vi "Main_v4.vi"() -> ()   [LabVIEW 2020]
uses:
  <userlib>/LevyLab/Relay Box/Type_defs/Resistor--enum.ctl
  <vilib>/Analysis/Matrix/Datatypes/RealMatrix.ctl
  subVIs/Global Variables.vi
  <vilib>/picture/3D Picture Control/Helpers/Apply Texture (no reference).vi
  <vilib>/picture/3D Picture Control/NI_3D Picture Control.lvlib
  <vilib>/Analysis/Matrix/NI_Matrix.lvlib
panel:
  in  "Run 2":bool=TRUE
  in  "Refresh Button":bool
  out "Ready?":bool
  in  "Done":bool
  in  "Help":bool
  in  "Abort":bool
  in  "Run":bool
  out "Estimated Time\nfor Lithography":timestamp=timestamp(-68372.87678205769 s since 1904-01-01) format="%<%H:%M:%S>T"
  in  "Visualization":T1(tab)
  out "Render":T2(plugin-control)
  out "Voltage Mapping":dbl(ramp)
  out "2D":T2(plugin-control)
  out "3D Picture":refnum<vi>(3d-picture)
  in  "Settings":T3(tab)
  in  "interpolation distance":dbl=0.1
  in  "Lithography Config File (.lcf)":path=path "c:/"
  in  "Patterns (drag-and-drop reorder)":i32(listbox)
  in  "image data max":dbl(slide)=100.0 min=0.0 max=100.0 scale=0.0..100.0
  in  "image data min":dbl(slide)=17.365269461077844 min=0.0 max=100.0 scale=0.0..100.0
  in  "AFM Type":u16(ring)=1 items=["Cypher", "MFP3D", "MFP3D_Lucy", "Simulation"]
  in  "Page":i32=1 min=0
  in  "Inkscape File (.svg)":path=path "c:/"
  in  "Background Image":path=path "c:/"
  # "Before you start the program\nchange these paths to the\ncorresponding files"
  # "In simulation mode, to change the perspective, hold the left button of mouse and drag in the picture.\nTo zoom in and out, hold the shift button, hold the left button of the mouse and drag up and down in\nthe picture."
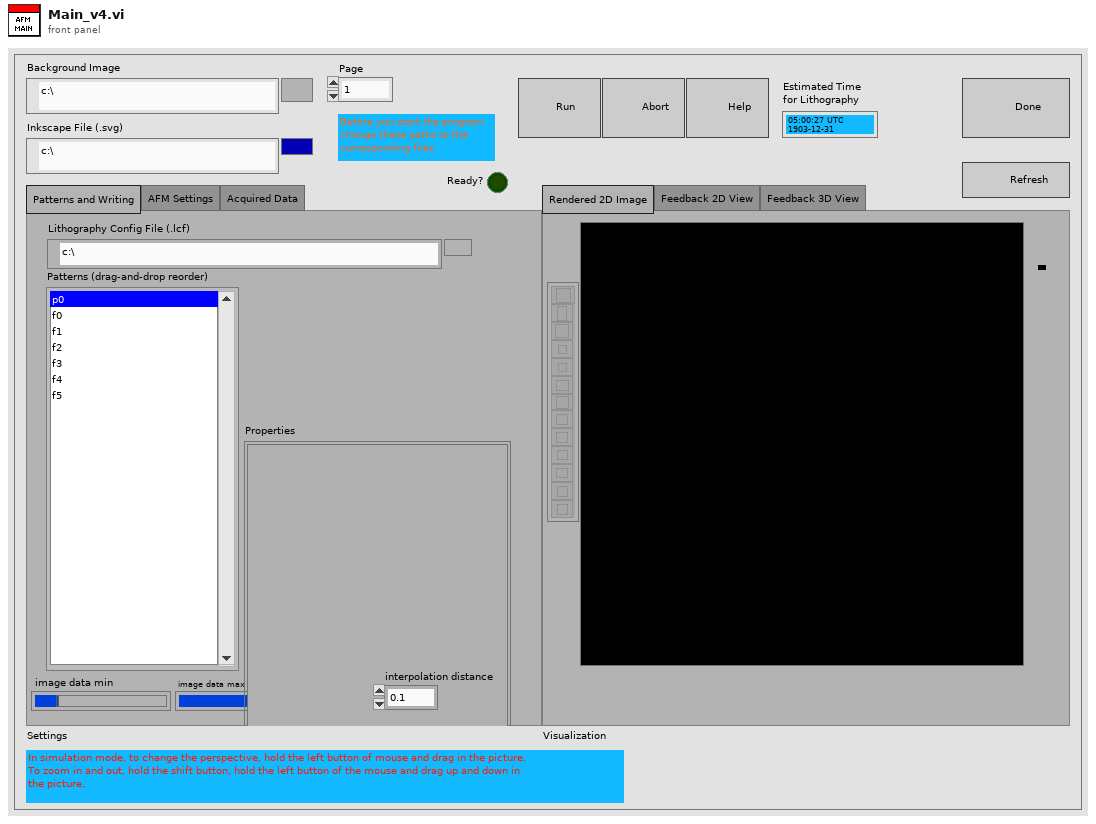
[diagram p1: front panel]
types:
  T1 = enum32{"Rendered 2D Image", "Feedback 2D View", "Feedback 3D View"}
  T2 = typedef "IMAQ Image.ctl" = refnum<image>
  T3 = enum32{"Patterns and Writing", "AFM Settings", "Acquired Data"}
  T4 = enum32{"invalid app kind", "Development System", "Run Time System", "Student Edition", "Embedded LabVIEW", "Evaluation", "Custom"}
  T5 = enum32{"Invalid", "Standard", "Closed", "Hidden", "Minimized", "Maximized"}
  T6 = typedef "Rectangle Properties - cluster.ctl" = cluster{"Enabled":bool, "Direction":u16, "Fill Orientation":u16, "Fill Spacing":dbl, "Speed (um/s)":T7, "Voltage (V)":T7, "Set Resistance":T10}
  T7 = typedef "Voltage - cluster.ctl" = cluster{"Schedule":T8, "Value":dbl, "Start Value":dbl, "End Value":dbl, "Min Value":dbl, "Max Value":dbl, "Duty Cycle (%)":dbl, "Signal Type":T9, "Cycle Number":dbl, "Phase (degrees)":dbl, "formula":string, "formula length (nm)":dbl, "formula resolution (nm)":dbl}
  T8 = typedef "Schedule - enum.ctl" = enum16{"Constant", "Ramp", "Fn. Generator", "Formula"}
  T9 = typedef "Signal Type - enum.ctl" = enum16{"Sine Wave", "Triangle Wave", "Square Wave", "Sawtooth Wave"}
  T10 = typedef "Resistor--enum.ctl" = enum16{"open", "discharge tip", "0 ohms", "100k ohm", "10M ohm", "1G ohm"}
  T11 = typedef "Funnel Properties - cluster.ctl" = cluster{"Enabled":bool, "Direction":u16, "Smooth Segments":dbl, "Bottom Segs.":dbl, "Speed (um/s)":T7, "Voltage (V)":T7, "Set Resistance":T10}
  T12 = typedef "Path Properties - cluster.ctl" = cluster{"Enabled":bool, "Direction":u16, "Fill Orientation":u16, "Smooth Segments":dbl, "Fill Spacing":dbl, "Speed (um/s)":T7, "Voltage (V)":T7, "Set Resistance":T10}
  T13 = cluster{"Path Properties":T12[], "Rectangle Properties":T6[], "Funnel Properties":T11[]}
  T14 = cluster{"SceneObject out":refnum<vi>, "Tip":refnum<vi>, "Canvas":refnum<vi>}
  T15 = typedef "imagedata.ctl" = cluster{"image type":i32, "image depth":i32, "image":u8[], "mask":u8[], "colors":u32[], "Rectangle":cluster{"left":i16, "top":i16, "right":i16, "bottom":i16}}
  T16 = typedef "NI_Matrix.lvlib/RealMatrix.ctl" = dbl[][]
  T17 = cluster{"Core":cluster{"Current VI Reference":refnum<vi>, "Close Panel on Exit?":bool}, "Parsing Data":cluster{"paths":cluster{"Fill Color":string, "Stroke Color":string, "Commands":cluster{"Command Type":string, "Coordinates":cluster{"X":dbl, "Y":dbl}[]}[], "Transformation Matrix 2":T16}[], "funnels":cluster{"Fill Color":string, "Stroke Color":string, "Commands":cluster{"Command Type":string, "Coordinates":cluster{"X":dbl, "Y":dbl}[]}[], "Transformation Matrix 2":T16}[], "rects":cluster{"Fill Color":string, "Stroke Color":string, "Width":dbl, "Height":dbl, "X":dbl, "Y":dbl, "Transformation Matrix":T16}[]}, "Lithography Data":cluster{"Name":string, "Litho":cluster{"X":dbl, "Y":dbl, "Speed":dbl, "Voltage":dbl}[], "Set Resistance":T10}[], "VI Refs":refnum<vi>[], "Data Queue":refnum<queue>, "3D":cluster{"SceneObject out":refnum<vi>, "Tip":refnum<vi>, "Canvas":refnum<vi>}}
  T18 = cluster{"paths":cluster{"Fill Color":string, "Stroke Color":string, "Commands":cluster{"Command Type":string, "Coordinates":cluster{"X":dbl, "Y":dbl}[]}[], "Transformation Matrix 2":T16}[], "funnels":cluster{"Fill Color":string, "Stroke Color":string, "Commands":cluster{"Command Type":string, "Coordinates":cluster{"X":dbl, "Y":dbl}[]}[], "Transformation Matrix 2":T16}[], "rects":cluster{"Fill Color":string, "Stroke Color":string, "Width":dbl, "Height":dbl, "X":dbl, "Y":dbl, "Transformation Matrix":T16}[]}
  T19 = cluster{"Name":string, "Litho":cluster{"X":dbl, "Y":dbl, "Speed":dbl, "Voltage":dbl}[], "Set Resistance":T10}[]
  T20 = cluster{"Current VI Reference":refnum<vi>, "Close Panel on Exit?":bool}
  T21 = cluster{"X":dbl, "Y":dbl, "Speed":dbl, "Voltage":dbl}
  T22 = cluster{" paths":cluster{"Fill Color":string, "Stroke Color":string, "Commands":cluster{"Command Type":string, "Coordinates":cluster{"X":dbl, "Y":dbl}[]}[], "Transformation Matrix 2":T16}[], " funnels":cluster{"Fill Color":string, "Stroke Color":string, "Commands":cluster{"Command Type":string, "Coordinates":cluster{"X":dbl, "Y":dbl}[]}[], "Transformation Matrix 2":T16}[], "rects":cluster{"Fill":string, "Stroke":string, "width":dbl, "height":dbl, "x":dbl, "y":dbl, "Transformation Matrix":T16}[]}
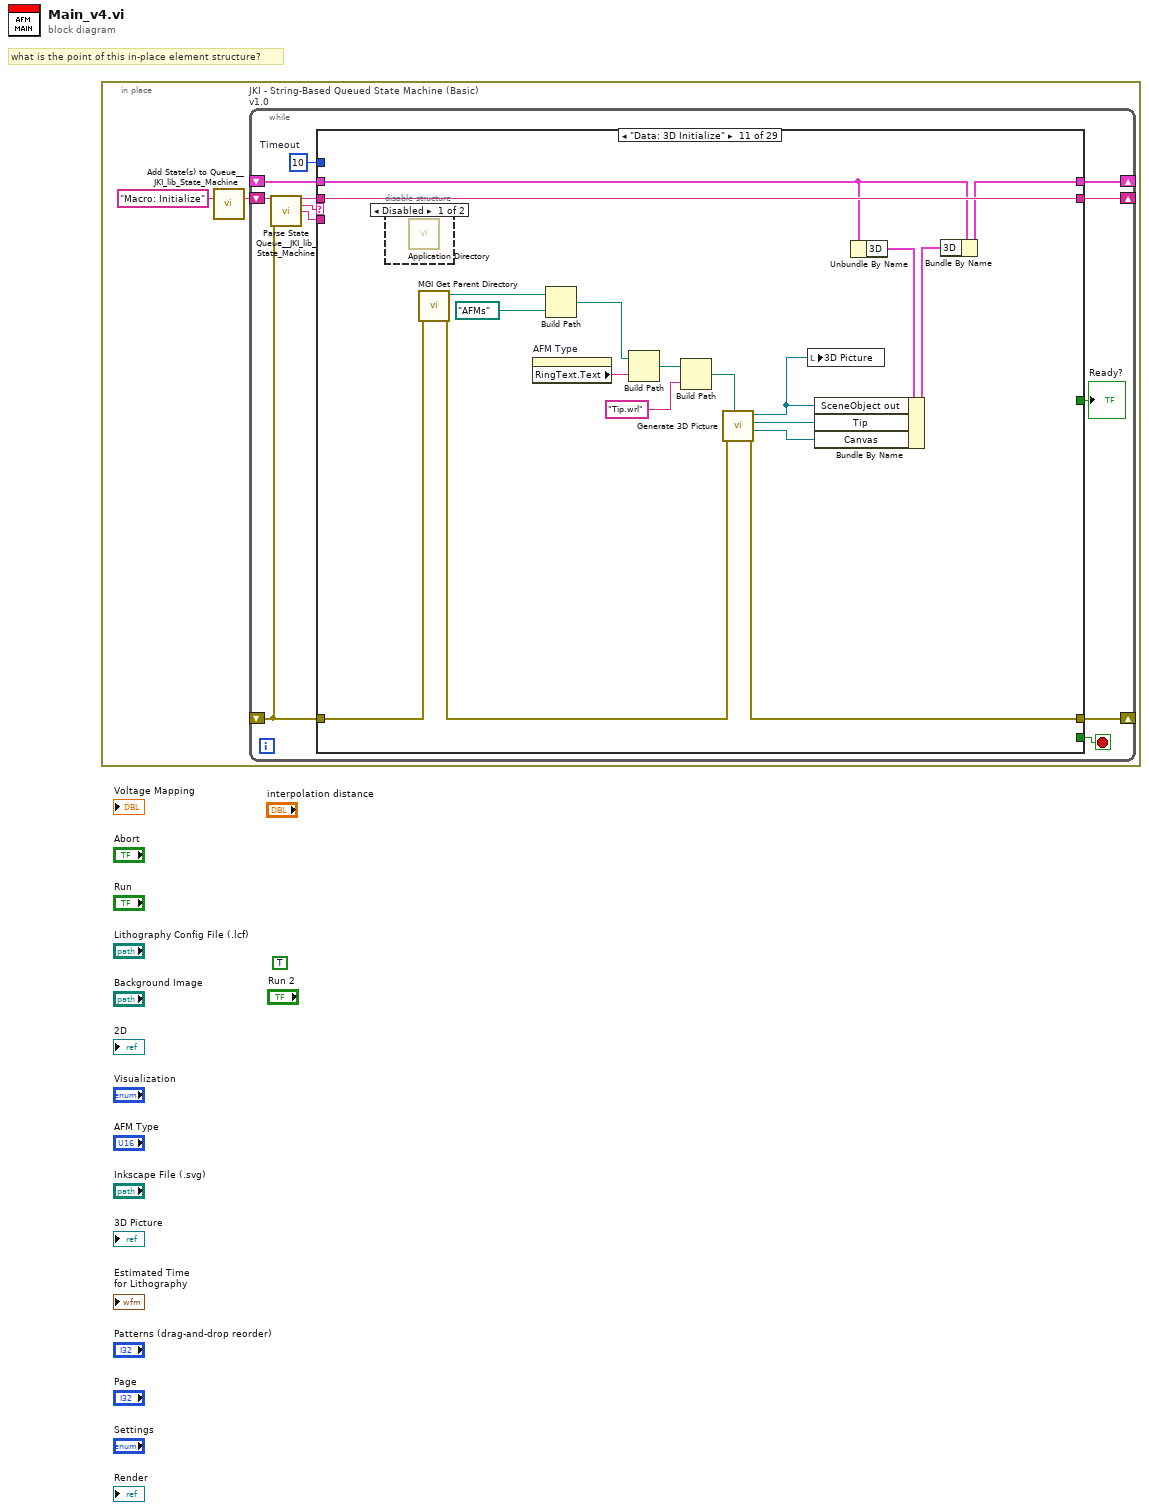
[diagram p0: block diagram]
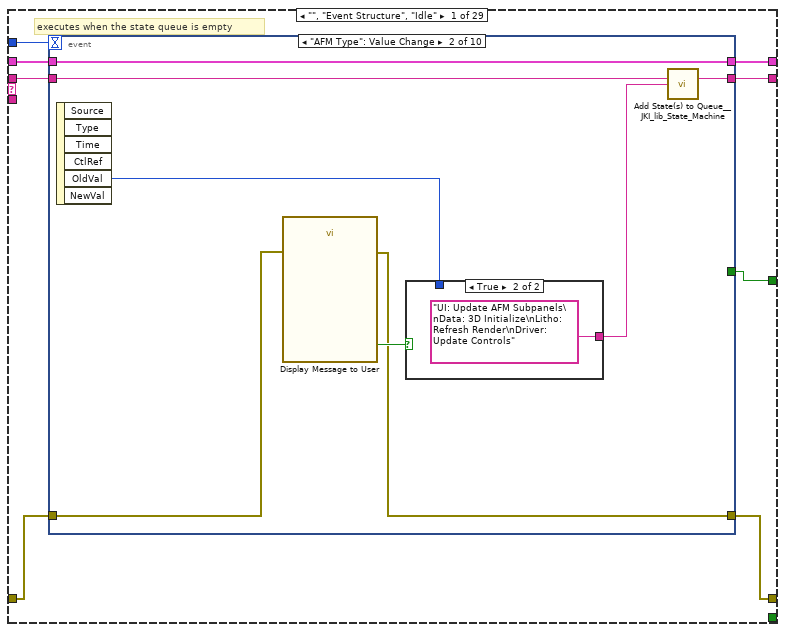
[diagram p2: hidden frame]
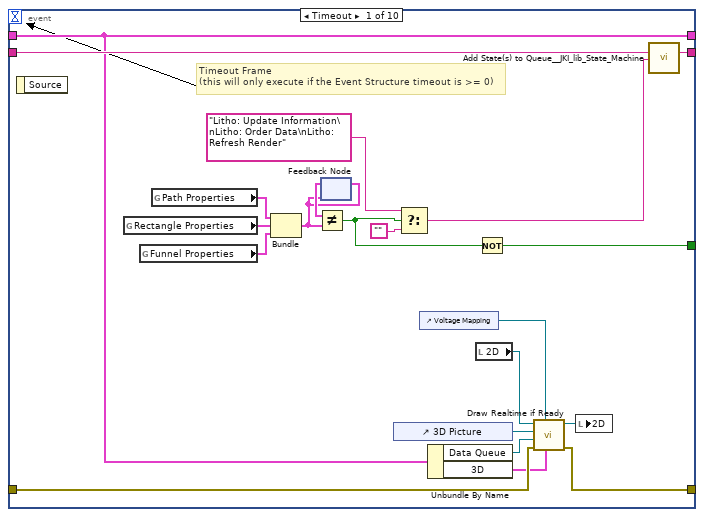
[diagram p3: hidden frame]
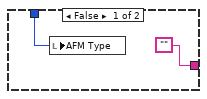
[diagram p4: hidden frame]
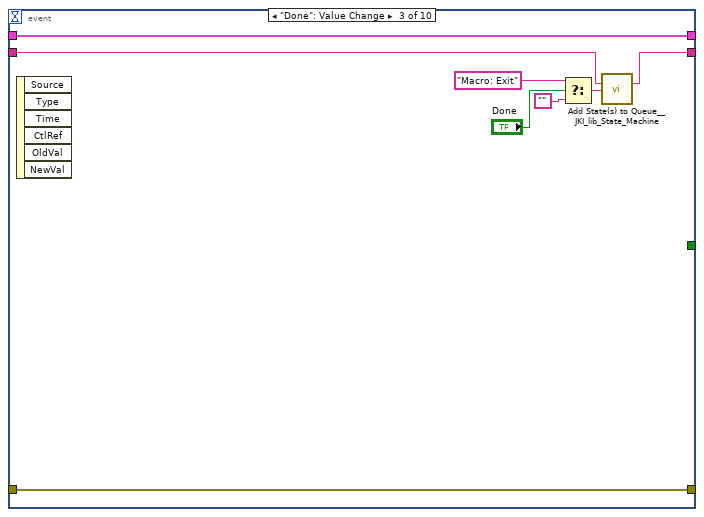
[diagram p5: hidden frame]
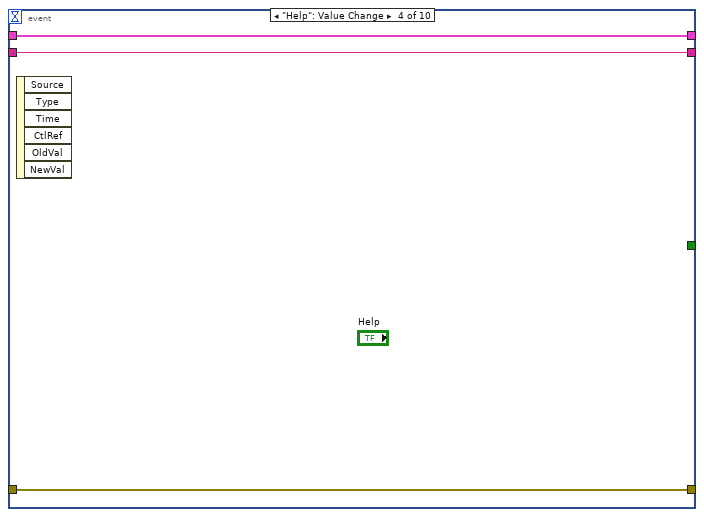
[diagram p6: hidden frame]
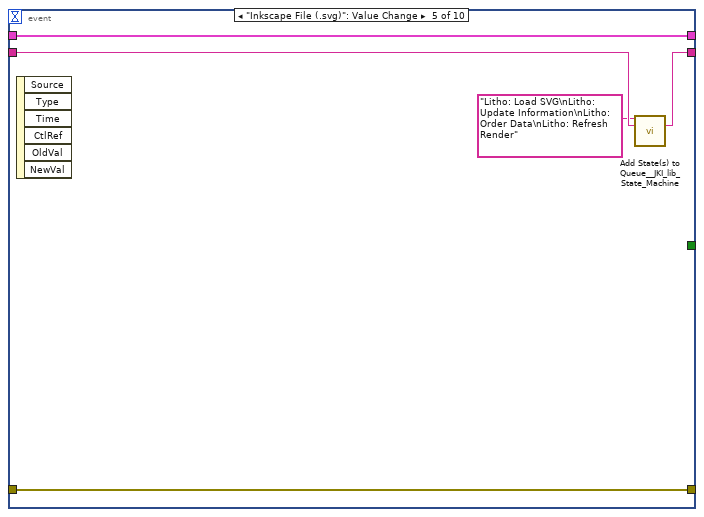
[diagram p7: hidden frame]
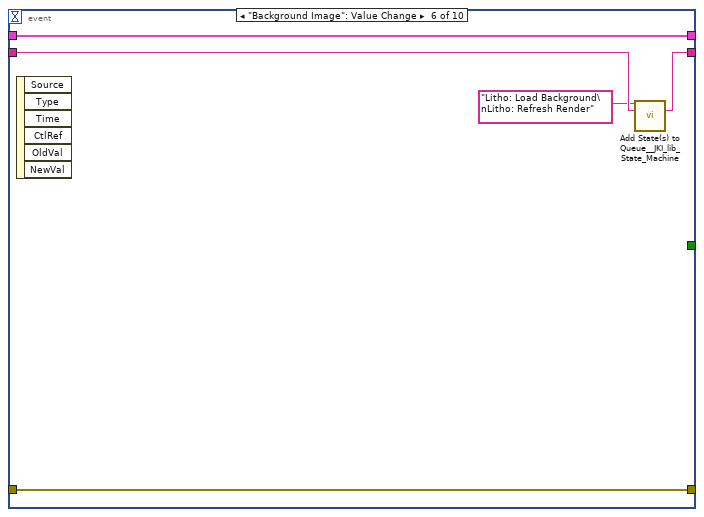
[diagram p8: hidden frame]
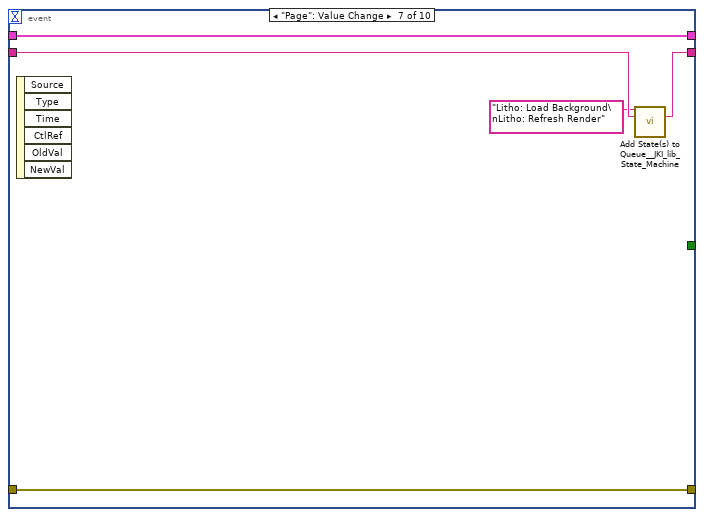
[diagram p9: hidden frame]
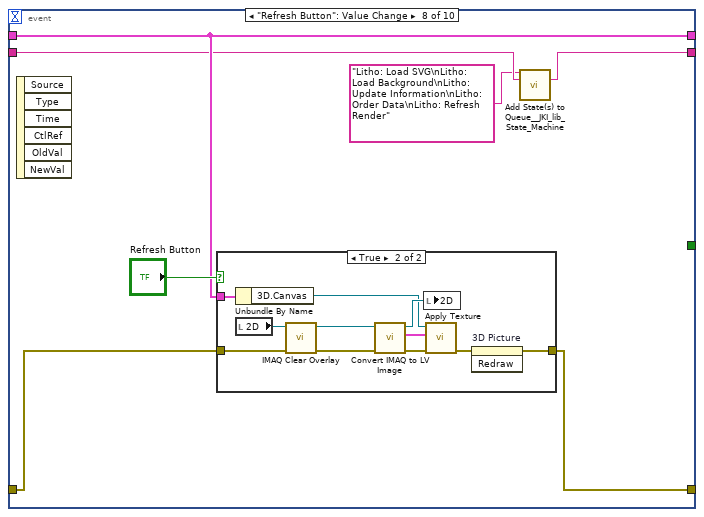
[diagram p10: hidden frame]
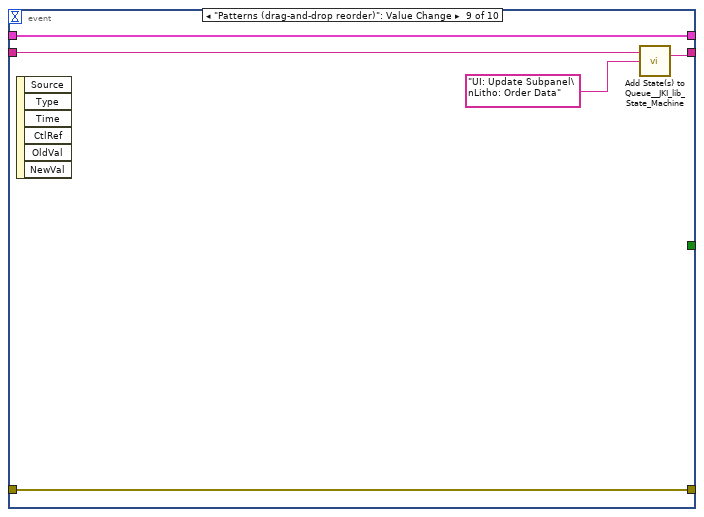
[diagram p12: hidden frame]
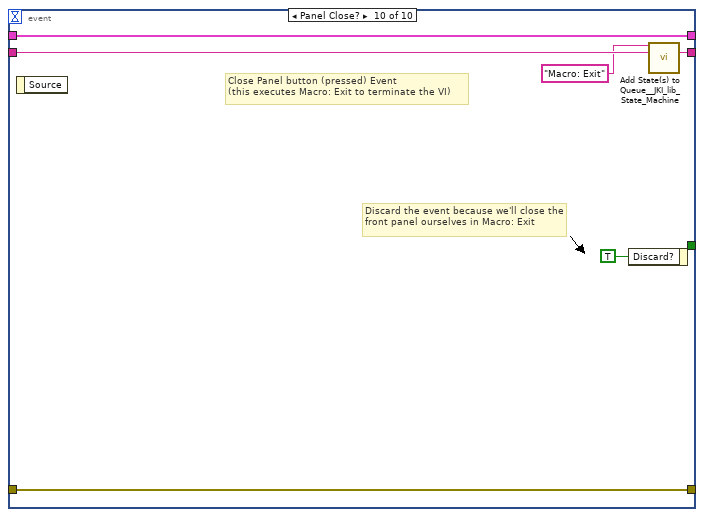
[diagram p13: hidden frame]
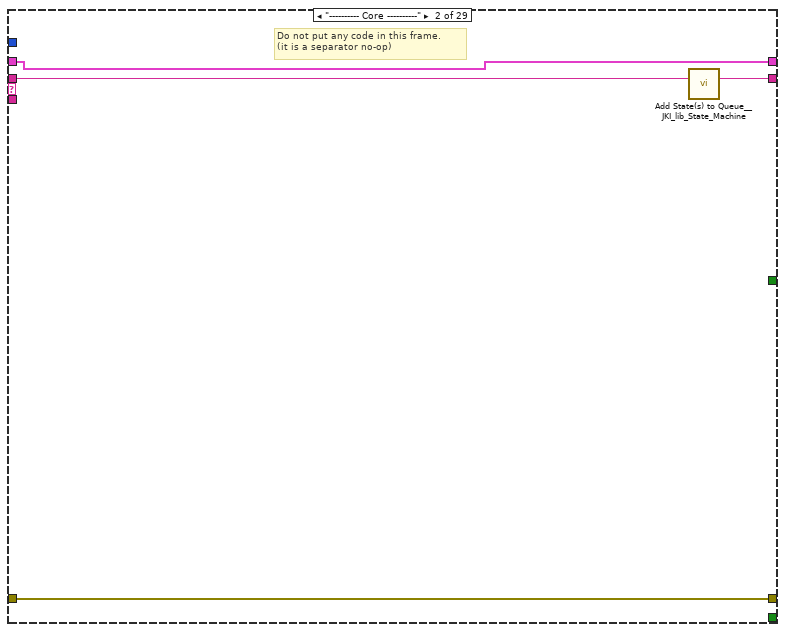
[diagram p14: hidden frame]
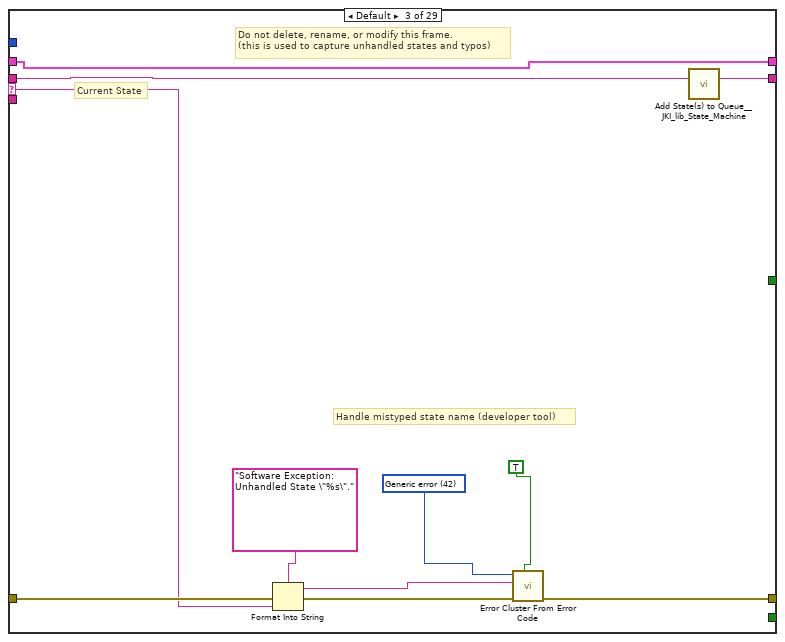
[diagram p15: hidden frame]
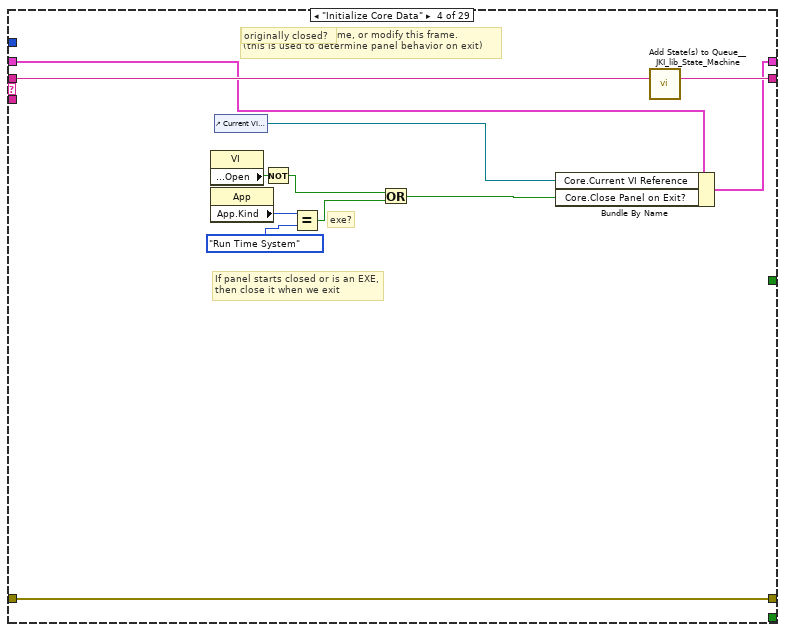
[diagram p16: hidden frame]
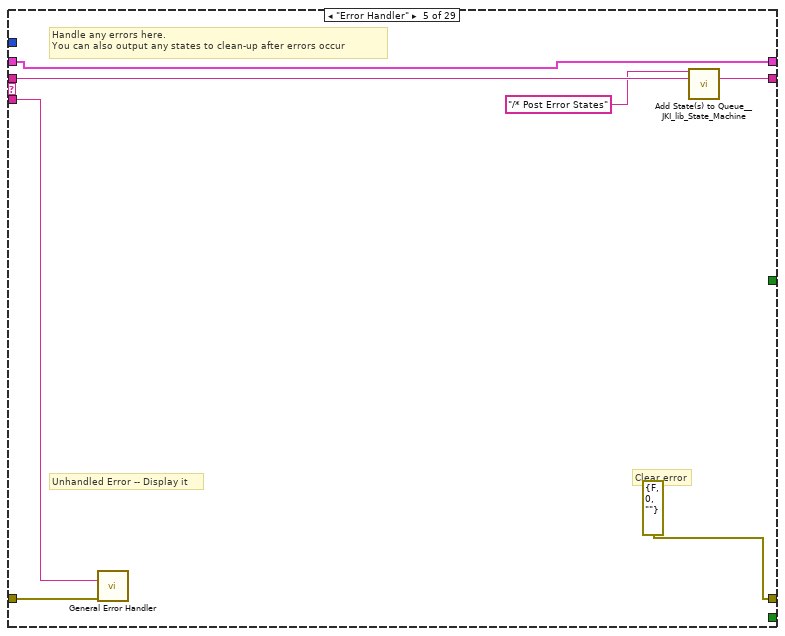
[diagram p17: hidden frame]
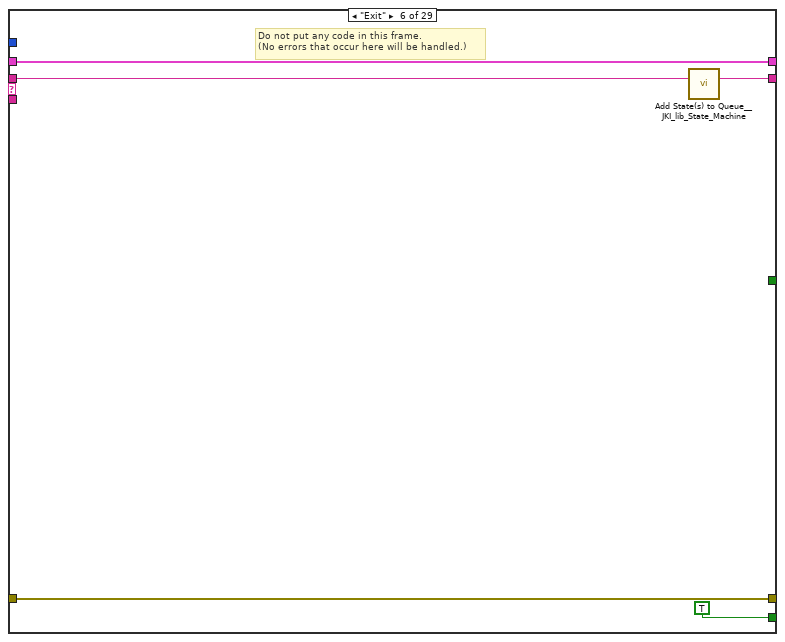
[diagram p18: hidden frame]
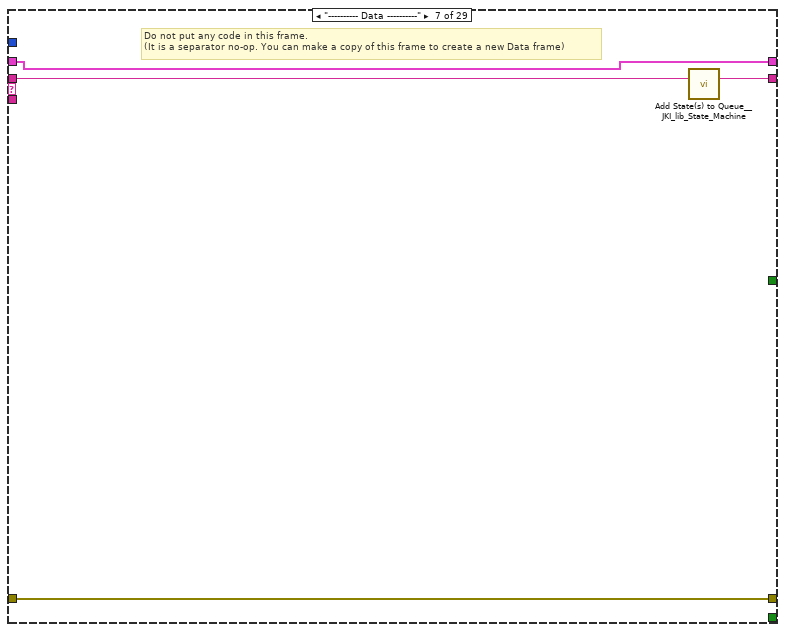
[diagram p19: hidden frame]
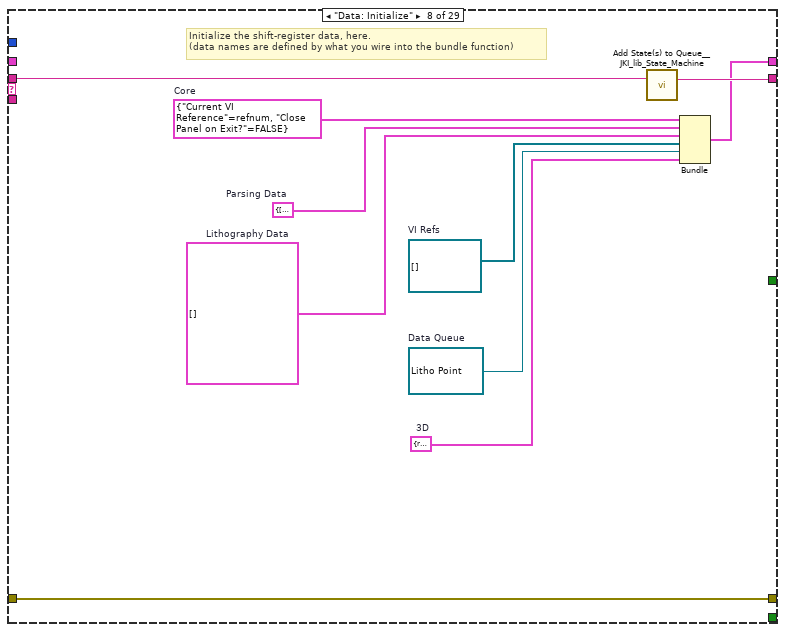
[diagram p20: hidden frame]
diagram:
  (unwired) TRUE
  # "what is the point of this in-place element structure?"
  n1 = in-place {
    n2 = call <vilib>:"Add State(s) to Queue__JKI_lib_State_Machine.vi"("State(s) in (\"\")"="Macro: Initialize") -> ("States Out"=w2:string)  [unwired: 14 in]
    n3 = while "JKI - String-Based Queued State Machine (Basic) v1.0" {
      shift-right: [w8] -> _
      shift-left: _ -> [w7]
      shift-right: [w3] -> _
      shift-left: _ -> [w4]
      shift-right: [w10] -> _
      shift-left: w2 -> [w11]
      stop <- w9 stop-if-true
      w6 = 10  # Timeout
      n4 = call <vilib>:"Parse State Queue__JKI_lib_State_Machine.vi"("State Queue"=w11, "Error In (no error)"=w4) -> ("Remaining States"=w13:string, "Current State"=w14:string, "Arguments"=w12:string)  [unwired: 11 in]
      n5 = case shown="\"Data: 3D Initialize\"" w14 {
        selector: w14 -> [_ _ w115 _ _ _ _ _ _ _ _ _ _ _ _ _ _ _ _ _ _ _ _ _ _ _ _ _ _]
        tunnel: w13 -> [w22 w114 w119 w137 w144 w149 w153 w161 w168 w187 w205 w222 w229 w243 w259 w277 w283 w294 w320 w325 w335 w339 w353 w380 w393 w410 w425 w429 w444]
        tunnel: w12 -> [_ _ _ _ w138 _ _ _ _ _ _ _ _ _ _ _ w280 w288 _ _ _ _ _ _ _ _ _ _ _]
        tunnel: w7 -> [w20 w111 w117 w128 w141 w145 w150 _ w167 w186 w194 w206 w226 w241 w250 w272 w281 w290 w317 w321 w326 w336 w349 w367 w388 w402 w413 w426 w437]
        tunnel: w4 -> [w19 w112 w120 w134 w140 w147 w151 w163 w169 w182 w190 w208 w227 w236 w251 w263 w279 w292 w318 w323 w333 w337 w344 w363 w399 w401 w414 w427 w435]
        tunnel: [w21 w113 w118 w136 w143 w148 w152 w160 w168 w187 w205 w221 w228 w242 w258 w276 w282 w293 w319 w324 w334 w338 w352 w379 w400 w409 w424 w428 w443] -> w10
        tunnel: [_ _ _ _ _ TRUE _ _ _ _ _ _ _ _ _ _ _ _ _ _ _ _ _ _ _ _ _ _ _] -> w9
        tunnel: [w18 w111 w117 w135 w141 w145 w150 w159 w165 w180 w197 w206 w226 w241 w250 w272 w281 w290 w317 w321 w326 w336 w347 w367 w394 w403 w413 w426 w437] -> w8
        tunnel: w6 -> [w17 _ _ _ _ _ _ _ _ _ _ _ _ _ _ _ _ _ _ _ _ _ _ _ _ _ _ _ _]
        tunnel: [w16 _ _ _ _ _ _ _ _ _ _ _ _ _ _ _ _ _ _ _ _ _ _ _ _ _ _ _ _] -> w5
        tunnel: [w15 w112 w121 w134 errorcluster {"status"=FALSE, "code"=0, "source"=""} ("error out") w147 w151 w163 w166 w181 w198 w207 w227 w238 w244 w271 w278 w291 w318 w323 w333 w337 w351 w372 w399 w405 w412 w427 w439] -> w3
        frame "", "Event Structure", "Idle" {
          # "executes when the state queue is empty"
          n6 = event shown="[1] \"AFM Type\": Value Change" {
            selector: _ -> [_ _ _ _ _ _ _ _ _ _]
            dyn-events: _ -> [_ _ _ _ _ _ _ _ _ _]
            timeout: w17 -> [_ _ _ _ _ _ _ _ _ _]
            tunnel: w22 -> [w43 w49 w59 w64 w70 w75 w80 w83 w103 w110]
            tunnel: [w42 w50 w60 w64 w69 w74 w79 w82 w102 w109] -> w21
            tunnel: w20 -> [w26 w51 w62 w65 w67 w72 w77 w84 w104 w107]
            tunnel: w19 -> [w30 w46 w61 w63 w68 w73 w78 w86 w101 w108]
            tunnel: [w26 w51 w62 w65 w67 w72 w77 w84 w104 w107] -> w18
            tunnel: [w24 _ _ _ _ _ _ _ _ _] -> w16
            tunnel: [w29 w44 w61 w63 w68 w73 w78 w85 w101 w108] -> w15
            event Timeout {
              # "Timeout Frame\n(this will only execute if the Event Structure timeout is >= 0)"
              n7 = event-data() -> ()  [unwired: 1 in, 1 out]
              n8 = global read "Global Variables.vi" "Rectangle Properties"() -> (w39:T6[])
              n9 = global read "Global Variables.vi" "Funnel Properties"() -> (w40:T11[])
              n10 = global read "Global Variables.vi" "Path Properties"() -> (w38:T12[])
              n11 = Bundle("Path Properties"=w38, "Rectangle Properties"=w39, "Funnel Properties"=w40) -> (w37:T13)  [unwired: 1 in]
              n12 = feedback #1(w37) -> (w41:T13)
              n13 = Not Equal?(x=w41, y=w37) -> (x != y?=w23:bool)
              n14 = feedback-in #1(w37) -> ()
              n15 = control-ref of="3D Picture"() -> (w32:refnum<vi>)
              n16 = Select(t="Litho: Update Information\nLitho: Order Data\nLitho: Refresh Render", s=w23, f="") -> (s? t:f=w34:string)
              n17 = control-ref of="Voltage Mapping"() -> (w33:refnum<vi>)
              n18 = Unbundle By Name(w26) -> ("Data Queue"=w28:refnum<queue>, "3D"=w27:T14)
              n19 = local read "2D"() -> (w31:T2)
              n20 = Not(x=w23) -> (.not. x?=w24:bool)
              n21 = call "Draw Realtime if Ready.vi"("3D"=w27, "Voltage Mapping"=w33, "error in (no error)"=w30, "Data Queue"=w28, "3D Picture"=w32, "Refnum in"=w31) -> ("error out"=w29:errorcluster, "Image out"=w25:T2)  [unwired: 4 in]
              n22 = local write "2D"(w25) -> ()
              n23 = call <vilib>:"Add State(s) to Queue__JKI_lib_State_Machine.vi"("State(s) in (\"\")"=w43, "State(s) at Back (\"\")"=w34) -> ("States Out"=w42:string)  [unwired: 13 in]
            }
            event "AFM Type": Value Change {
              n24 = event-data() -> ("OldVal"=w47:u16)  [unwired: 1 in, 5 out]
              n25 = call "Display Message to User"("error in (no error)"=w46) -> ("error out"=w44:errorcluster, "OK"=w48:bool)  [unwired: 9 in]
              n26 = case shown="True" w48 {
                tunnel: ["" "UI: Update AFM Subpanels\nData: 3D Initialize\nLitho: Refresh Render\nDriver: Update Controls" ("State(s) at Back (\"\")")] -> w45
                tunnel: w47 -> [w52 _]
                frame False {
                  n27 = local write "AFM Type"(w52) -> ()
                }
                frame True {
                }
              }
              n28 = call <vilib>:"Add State(s) to Queue__JKI_lib_State_Machine.vi"("State(s) in (\"\")"=w49, "State(s) at Back (\"\")"=w45) -> ("States Out"=w50:string)  [unwired: 13 in]
            }
            event "Done": Value Change {
              n29 = event-data() -> ()  [unwired: 1 in, 6 out]
              n30 = Select(t="Macro: Exit", s="Done", f="") -> (s? t:f=w55:string)
              n31 = call <vilib>:"Add State(s) to Queue__JKI_lib_State_Machine.vi"("State(s) in (\"\")"=w59, "State(s) at Back (\"\")"=w55) -> ("States Out"=w60:string)  [unwired: 13 in]
            }
            event "Help": Value Change {
              n32 = event-data() -> ()  [unwired: 1 in, 6 out]
            }
            event "Inkscape File (.svg)": Value Change {
              n33 = event-data() -> ()  [unwired: 1 in, 6 out]
              n34 = call <vilib>:"Add State(s) to Queue__JKI_lib_State_Machine.vi"("State(s) in Front (\"\")"="Litho: Load SVG\nLitho: Update Information\nLitho: Order Data\nLitho: Refresh Render", "State(s) in (\"\")"=w70) -> ("States Out"=w69:string)  [unwired: 13 in]
            }
            event "Background Image": Value Change {
              n35 = event-data() -> ()  [unwired: 1 in, 6 out]
              n36 = call <vilib>:"Add State(s) to Queue__JKI_lib_State_Machine.vi"("State(s) in Front (\"\")"="Litho: Load Background\nLitho: Refresh Render", "State(s) in (\"\")"=w75) -> ("States Out"=w74:string)  [unwired: 13 in]
            }
            event "Page": Value Change {
              n37 = event-data() -> ()  [unwired: 1 in, 6 out]
              n38 = call <vilib>:"Add State(s) to Queue__JKI_lib_State_Machine.vi"("State(s) in Front (\"\")"="Litho: Load Background\nLitho: Refresh Render", "State(s) in (\"\")"=w80) -> ("States Out"=w79:string)  [unwired: 13 in]
            }
            event "Refresh Button": Value Change {
              n39 = event-data() -> ()  [unwired: 1 in, 6 out]
              n40 = case shown="True" "Refresh Button" {
                tunnel: w86 -> [w88 w98]
                tunnel: [w88 w91] -> w85
                tunnel: w84 -> [_ w90]
                frame False {
                }
                frame True {
                  n41 = Unbundle By Name(w90) -> ("3D.Canvas"=w89:refnum<vi>)
                  n42 = local read "2D"() -> (w99:T2)
                  n43 = call "IMAQ Clear Overlay"("error in (no error)"=w98, "Image"=w99) -> ("error out"=w94:errorcluster, "Image Out"=w93:T2)  [unwired: 8 in]
                  n44 = call "Convert IMAQ to LV Image.vi"("error in (no error)"=w94, "IMAQImage In (RGB 32)"=w93) -> ("error out"=w95:errorcluster, "Output Image"=w96:T15, "IMAQImage Out"=w92:T2)  [unwired: 7 in]
                  n45 = local write "2D"(w92) -> ()
                  n46 = call-poly <vilib>:"Apply Texture.vi"("error in (no error)"=w95, "Image Data"=w96, "Scene Object In"=w89) -> ("error out"=w97:errorcluster)  [unwired: 7 in, 1 out]
                  n47 = invoke on="3D Picture" class="SceneGraphDisp (strict)" method="Redraw"(error in=w97) -> (error out=w91:errorcluster)  [unwired: 2 in, 2 out]
                }
              }
              n48 = call <vilib>:"Add State(s) to Queue__JKI_lib_State_Machine.vi"("State(s) in Front (\"\")"="Litho: Load SVG\nLitho: Load Background\nLitho: Update Information\nLitho: Order Data\nLitho: Refresh Render", "State(s) in (\"\")"=w83) -> ("States Out"=w82:string)  [unwired: 13 in]
            }
            event "Patterns (drag-and-drop reorder)": Value Change {
              n49 = event-data() -> ()  [unwired: 1 in, 6 out]
              n50 = call <vilib>:"Add State(s) to Queue__JKI_lib_State_Machine.vi"("State(s) in (\"\")"=w103, "State(s) at Back (\"\")"="UI: Update Subpanel\nLitho: Order Data" ("State(s) at Back (\"\")")) -> ("States Out"=w102:string)  [unwired: 13 in]
            }
            event Panel Close? {
              # "Discard the event because we'll close the front panel ourselves in Macro: Exit"
              # "Close Panel button (pressed) Event\n(this executes Macro: Exit to terminate the VI)"
              n51 = event-data() -> ()  [unwired: 1 in, 1 out]
              n52 = event-data("Discard?"=TRUE) -> ()  [unwired: 1 in, 1 out]
              n53 = call <vilib>:"Add State(s) to Queue__JKI_lib_State_Machine.vi"("State(s) in Front (\"\")"="Macro: Exit", "State(s) in (\"\")"=w110) -> ("States Out"=w109:string)  [unwired: 13 in]
            }
          }
        }
        frame "---------- Core ----------" {
          # "Do not put any code in this frame.\n(it is a separator no-op)"
          n54 = call <vilib>:"Add State(s) to Queue__JKI_lib_State_Machine.vi"("State(s) in (\"\")"=w114) -> ("States Out"=w113:string)  [unwired: 14 in]
        }
        frame Default {
          w124 = 42 items=["No error", "Argument error", "Memory is full", "Out of zone", "End of file", "File already open", "Generic file I/O error", "File not found", "File permission error", "Disk is full", "Duplicate path", "Too many files open", "System feature not enabled", "Resource file not found", "Cannot add resource", "Resource not found", "Image not found", "Image memory error", "Pen does not exist", "Config type invalid", "Config token not found", "Config parse error", "Config memory error", "Bad external code format", "Bad external code offset", "External code not present", "Null window", "Destroy window error", "Null menu", "Print aborted", "Bad print record", "Print driver error", "Windows error during printing", "Memory error during printing", "Print dialog error", "Generic print error", "Invalid device refnum", "Device not found", "Device parameter error", "Device unit error", "Cannot open device", "Device call aborted", "Generic error", "Cancelled by user", "Object ID too low", "Object ID too high", "Object not in heap", "Unknown heap", "Unknown object (invalid DefProc)", "Unknown object (DefProc not in table)", "Message out of range", "Invalid (null) method", "Unknown message", "Manager call not supported", "Bad address", "Network operation in progress", "Network operation timed out", "Connection is busy", "Network attribute not supported", "Network error", "Address in use", "System out of memory", "Connection aborted", "Connection refused", "Not connected", "Already connected", "Connection closed", "Initialization error (interapplication manager)", "Bad occurrence", "Wait on unbound occurrence handler", "Occurrence queue overflow", "Datalog type conflict", "Unused", "Unrecognized type (interapplication manager)", "Memory corrupt", "Failed to make temporary DLL", "Old CIN version", "Drag socket not found", "Failed to load drop-object", "Failed to register OLE object", "Failed to release OLE object", "Format specifier type mismatch", "Unknown format specifier", "Too few format specifiers", "Too many format specifiers", "Scan failed", "Newer CIN version", "Error converting to variant", "Runtime menu error", "Password tampered", "Variant attribute not found", "Incompatible variant data type", "Event data is not available", "Event Store is not present", "Occurrence is not found", "Event Queue is not created", "Event info is not available", "Refnum passed is NULL", "Error retrieving Class GUID", "Error retrieving CoClass GUID", "Error retrieving TypeLib GUID.", "Bad built application magic bytes.", "Specific driver is different from the specific driver associated with the Logical Name.", "There is no session opened to the class driver.", "Max Error", "MAX - Error with config objects", "MAX - Error loading configuration", "MAX - Group not supported"]
          # "Current State"
          # "Do not delete, rename, or modify this frame.\n(this is used to capture unhandled states and typos)"
          # "Handle mistyped state name (developer tool)"
          n55 = Format Into String(format string="Software Exception: Unhandled State \"%s\"." ("message"), error in=w120, w115) -> (resulting string=w123:string, error out=w122:errorcluster)  [unwired: 1 in]
          n56 = call <vilib>:"Error Cluster From Error Code.vi"("show call chain? (False)"=TRUE, "error in (no error)"=w122, "error message (\"\")"=w123, "error code (0)"=w124) -> ("error out"=w121:errorcluster)  [unwired: 5 in]
          n57 = call <vilib>:"Add State(s) to Queue__JKI_lib_State_Machine.vi"("State(s) in (\"\")"=w119) -> ("States Out"=w118:string)  [unwired: 14 in]
        }
        frame "Initialize Core Data" {
          # "Do not delete, rename, or modify this frame.\n(this is used to determine panel behavior on exit)"
          # "originally closed?"
          # "exe?"
          # "If panel starts closed or is an EXE, then close it when we exit"
          n58 = property class="VI"() -> ("Front Panel.Open"=w133:bool)  [unwired: 2 in, 2 out]
          n59 = property class="App"() -> ("App.Kind"=w132:T4)  [unwired: 2 in, 2 out]
          n60 = control-ref of="Current VI Reference"() -> (w126:refnum<vi>)
          n61 = Not(x=w133) -> (.not. x?=w130:bool)
          n62 = Equal?(x=w132, y=T4."Run Time System" ("Application:Kind")) -> (x = y?=w129:bool)
          n63 = Or(x=w130, y=w129) -> (x .or. y?=w127:bool)
          n64 = Bundle By Name(cluster=w128, "Core.Current VI Reference"=w126, "Core.Close Panel on Exit?"=w127) -> (w135:T17)
          n65 = call <vilib>:"Add State(s) to Queue__JKI_lib_State_Machine.vi"("State(s) in (\"\")"=w137) -> ("States Out"=w136:string)  [unwired: 14 in]
        }
        frame "Error Handler" {
          # "Unhandled Error -- Display it"
          # "Handle any errors here.\nYou can also output any states to clean-up after errors occur"
          # "Clear error"
          n66 = call <vilib>:"General Error Handler.vi"("[error source] (\" \")"=w138, "error in (no error)"=w140) -> ()  [unwired: 9 in, 5 out]
          n67 = call <vilib>:"Add State(s) to Queue__JKI_lib_State_Machine.vi"("State(s) in Front (\"\")"="/* Post Error States", "State(s) in (\"\")"=w144) -> ("States Out"=w143:string)  [unwired: 13 in]
        }
        frame "Exit" {
          # "Do not put any code in this frame.\n(No errors that occur here will be handled.)"
          n68 = call <vilib>:"Add State(s) to Queue__JKI_lib_State_Machine.vi"("State(s) in (\"\")"=w149) -> ("States Out"=w148:string)  [unwired: 14 in]
        }
        frame "---------- Data ----------" {
          # "Do not put any code in this frame.\n(It is a separator no-op. You can make a copy of this frame to create a new Data frame)"
          n69 = call <vilib>:"Add State(s) to Queue__JKI_lib_State_Machine.vi"("State(s) in (\"\")"=w153) -> ("States Out"=w152:string)  [unwired: 14 in]
        }
        frame "Data: Initialize" {
          w154 = T18 {"paths"=[], "funnels"=[], "rects"=[]}  # Parsing Data
          w157 = refnum<queue> refnum  # Data Queue
          w158 = T14 {"SceneObject out"=refnum, "Tip"=refnum, "Canvas"=refnum}  # 3D
          w156 = refnum<vi>[] []  # VI Refs
          w155 = T19 []  # Lithography Data
          w162 = T20 {"Current VI Reference"=refnum, "Close Panel on Exit?"=FALSE}  # Core
          # "Initialize the shift-register data, here.\n(data names are defined by what you wire into the bundle function)"
          n70 = call <vilib>:"Add State(s) to Queue__JKI_lib_State_Machine.vi"("State(s) in (\"\")"=w161) -> ("States Out"=w160:string)  [unwired: 14 in]
          n71 = Bundle("Core"=w162, "Parsing Data"=w154, "Lithography Data"=w155, "VI Refs"=w156, "Data Queue"=w157, "3D"=w158) -> (w159:T17)  [unwired: 1 in]
        }
        frame "Data: Run Edit VIs" {
          w170 = path[] [path "subVIs/subpanel/Path Edit.vi", path "subVIs/subpanel/Rect Edit.vi", path "subVIs/subpanel/Funnel Edit.vi"]  # Edit VIs
          n72 = for {
            tunnel: [w174] -> w164 mode=indexing
            shift-right: [w172] -> w166
            shift-left: w169 -> [w173]
            tunnel: w170 -> [w171] mode=indexing
            # "Load and run Plugin VIs"
            n73 = Open VI Reference(vi path=w171, error in (no error)=w173) -> (vi reference=w175:refnum<vi>, error out=w176:errorcluster)  [unwired: 4 in]
            n74 = invoke class="VI" method="Run VI"(reference=w175, error in=w176, "Wait until done"=FALSE ("Wait Until Done")) -> (reference out=w174:refnum<vi>, error out=w172:errorcluster)  [unwired: 2 in, 3 out]
          }
          n75 = Bundle By Name(cluster=w167, "VI Refs"=w164) -> (w165:T17)
        }
        frame "Data: Create Data Queue" {
          w178 = T21 {"X"=0.0, "Y"=0.0, "Speed"=0.0, "Voltage"=0.0}  # Litho Point
          n76 = Obtain Queue(name (unnamed)="Litho Data", element data type=w178, error in (no error)=w182) -> (queue out=w185:refnum<queue>, error out=w184:errorcluster)  [unwired: 2 in, 1 out]
          n77 = Flush Queue(queue=w185, error in (no error)=w184) -> (queue out=w183:refnum<queue>, error out=w181:errorcluster)  [unwired: 1 out]
          n78 = Bundle By Name(cluster=w186, "Data Queue"=w183) -> (w180:T17)
        }
        frame "Data: 3D Initialize" {
          n79 = disable-structure shown="Disabled" {
            frame Disabled {
              n80 = call <vilib>:"Application Directory.vi"() -> ()  [unwired: 1 out]
            }
            frame Enabled {
            }
          }
          n81 = call <userlib>:"MGI Get Parent Directory.vi"("Error In"=w190) -> ("Error Out"=w189:errorcluster, "Parent Directory"=w188:path)  [unwired: 9 in]
          n82 = property on="AFM Type" class="Ring (strict)"() -> ("RingText.Text"=w204:string)  [unwired: 2 in, 2 out]
          n83 = Build Path(base path=w188, name or relative path=path "AFMs" ("path")) -> (appended path=w196:path)
          n84 = Build Path(base path=w196, name or relative path=w204) -> (appended path=w203:path)
          n85 = Build Path(base path=w203, name or relative path="Tip.wrl") -> (appended path=w191:path)
          n86 = call "Generate 3D Picture.vi"("Tip Model File (.wrl)"=w191, "error in (no error)"=w189) -> ("error out"=w198:errorcluster, "Canvas"=w202:refnum<vi>, "Tip"=w201:refnum<vi>, "SceneObject out"=w192:refnum<vi>)  [unwired: 6 in]
          n87 = local write "3D Picture"(w192) -> ()
          n88 = Unbundle By Name(w194) -> ("3D"=w193:T14)
          n89 = Bundle By Name(cluster=w193, "SceneObject out"=w192, "Tip"=w201, "Canvas"=w202) -> (w200:T14)
          n90 = Bundle By Name(cluster=w194, "3D"=w200) -> (w197:T17)
        }
        frame "Data: Cleanup" {
          # "Cleanup any data and references, here.\n(this is called automatically, by the Macro: Exit)"
          n91 = Unbundle By Name(w206) -> ("Core.Current VI Reference"=w219:refnum<vi>, "VI Refs"=w220:refnum<vi>[], "Data Queue"=w218:refnum<queue>)
          n92 = property on="Acquired Data" class="SubPnl"() -> ("InsertedVI"=w215:refnum<vi>)  [unwired: 2 in, 2 out]
          n93 = call "Abort If Not Refnum.vi"("error in (no error)"=w208, "VI in"=w215) -> ("error out"=w212:errorcluster)  [unwired: 9 in]
          n94 = invoke on="Acquired Data" class="SubPnl" method="Remove VI"(error in=w212) -> (error out=w211:errorcluster)  [unwired: 2 in, 2 out]
          n95 = property on="AFM Settings" class="SubPnl"() -> ("InsertedVI"=w214:refnum<vi>)  [unwired: 2 in, 2 out]
          n96 = call "Abort If Not Refnum.vi"("error in (no error)"=w211, "VI in"=w214) -> ("error out"=w213:errorcluster)  [unwired: 9 in]
          n97 = invoke on="AFM Settings" class="SubPnl" method="Remove VI"(error in=w213) -> (error out=w210:errorcluster)  [unwired: 2 in, 2 out]
          n98 = for {
            tunnel: w220 -> [w225] mode=indexing
            shift-right: [w223] -> w217
            shift-left: w210 -> [w224]
            n99 = call "Abort If Not Refnum.vi"("error in (no error)"=w224, "VI in"=w225) -> ("error out"=w223:errorcluster)  [unwired: 9 in]
          }
          n100 = Release Queue(queue=w218, force destroy? (F)=TRUE, error in (no error)=w217) -> (error out=w216:errorcluster)  [unwired: 2 out]
          n101 = Close Reference(reference=w219, error in (no error)=w216) -> (error out=w207:errorcluster)
          n102 = call <vilib>:"Add State(s) to Queue__JKI_lib_State_Machine.vi"("State(s) in (\"\")"=w222) -> ("States Out"=w221:string)  [unwired: 14 in]
        }
        frame "---------- UI ----------" {
          # "Do not put any code in this frame.\n(It is a separator no-op. You can make a copy of this frame to create a new UI frame)"
          n103 = call <vilib>:"Add State(s) to Queue__JKI_lib_State_Machine.vi"("State(s) in (\"\")"=w229) -> ("States Out"=w228:string)  [unwired: 14 in]
        }
        frame "UI: Initialize" {
          # "populate AFM Type ring"
          # "resize front panel"
          # "FIX THIS TO IGNORE .svn"
          # "Initialize the User Interface, here.\n(this is called automatically, by the Macro: Init)"
          n104 = call <userlib>:"Fit VI window to Largest Dec__ogtk.vi"("error in (no error)"=w236) -> ("error out"=w233:errorcluster)  [unwired: 5 in, 1 out]
          n105 = disable-structure shown="Disabled" {
            frame Disabled {
              n106 = call <vilib>:"Application Directory.vi"() -> ()  [unwired: 1 out]
            }
            frame Enabled {
            }
          }
          n107 = call <userlib>:"MGI Get Parent Directory.vi"("Error In"=w233) -> ("Error Out"=w232:errorcluster, "Parent Directory"=w231:path)  [unwired: 9 in]
          n108 = Build Path(base path=w231, name or relative path="AFMs" ("path")) -> (appended path=w239:path)
          n109 = List Folder(path=w239, error in=w232) -> (folder names=w237:string[], error out=w230:errorcluster)  [unwired: 2 in, 2 out]
          n110 = Array Subset(array=w237, index=0) -> (w235:string[])  [unwired: 1 in]
          n111 = property on="AFM Type" class="Ring (strict)"(error in=w230, "Strings []"=w235) -> (error out=w238:errorcluster)  [unwired: 1 in, 1 out]
          n112 = call <vilib>:"Add State(s) to Queue__JKI_lib_State_Machine.vi"("State(s) in (\"\")"=w243) -> ("States Out"=w242:string)  [unwired: 14 in]
        }
        frame "UI: Update Subpanel" {
          # "Subpanel is updated to reflect pattern's type."
          n113 = Unbundle By Name(w250) -> ("VI Refs"=w246:refnum<vi>[])
          n114 = control-ref of="Patterns (drag-and-drop reorder)"() -> (w257:refnum<vi>)
          n115 = call "Get Selected Pattern.vi"("error in (no error)"=w251, "ListBox in"=w257) -> ("error out"=w253:errorcluster, "Pattern Index"=w247:i32, "Type"=w256:string)  [unwired: 7 in]
          n116 = case shown="\"f\", Default" w256 {
            tunnel: [2 0 1] -> w255
            frame "f", Default {
            }
            frame "p" {
            }
            frame "r" {
            }
          }
          n117 = Index Array(array=w246, index=w255) -> (element=w245:refnum<vi>)
          n118 = invoke class="VI" method="Ctrl Val.Set"(reference=w245, error in=w253, "Control Name"="Index", "Value"=w247) -> (reference out=w248:refnum<vi>, error out=w254:errorcluster)  [unwired: 1 in, 3 out]
          n119 = invoke on="Properties" class="SubPanel" method="Remove VI"(error in=w254) -> (error out=w249:errorcluster)  [unwired: 2 in, 2 out]
          n120 = invoke on="Properties" class="SubPanel" method="Insert VI"(error in=w249, "VI Ref"=w248) -> (error out=w244:errorcluster)  [unwired: 2 in, 3 out]
          n121 = call <vilib>:"Add State(s) to Queue__JKI_lib_State_Machine.vi"("State(s) in (\"\")"=w259) -> ("States Out"=w258:string)  [unwired: 14 in]
        }
        frame "UI: Update AFM Subpanels" {
          # "data cluster should not be going into subVIs!"
          # "Subpanels are updated to reflect AFM type."
          n122 = control-ref of="Background Image"() -> (w266:refnum<vi>)
          n123 = control-ref of="AFM Type"() -> (w274:refnum<vi>)
          n124 = control-ref of="Inkscape File (.svg)"() -> (w273:refnum<vi>)
          n125 = control-ref of="AFM Settings"() -> (w264:refnum<vi>)
          n126 = control-ref of="Acquired Data"() -> (w268:refnum<vi>)
          n127 = control-ref of="Run"() -> (w267:refnum<vi>)
          n128 = control-ref of="Abort"() -> (w269:refnum<vi>)
          n129 = call "Load AFM Subpanel.vi"("Ring in"=w274, "Background Image"=w266, "name or relative path"="Driver.vi", "Inkscape File (.svg)"=w273, "input cluster"=w272, "Subpanel"=w264, "error in (no error)"=w263, "Run"=w267, "Abort"=w269) -> ("error out"=w275:errorcluster)  [unwired: 5 in, 1 out]
          n130 = call "Load AFM Subpanel.vi"("Ring in"=w274, "Background Image"=w266, "name or relative path"="Acquired Data.vi", "Inkscape File (.svg)"=w273, "input cluster"=w272, "Subpanel"=w268, "error in (no error)"=w275, "Run"=w267, "Abort"=w269) -> ("error out"=w271:errorcluster)  [unwired: 5 in, 1 out]
          n131 = call <vilib>:"Add State(s) to Queue__JKI_lib_State_Machine.vi"("State(s) in (\"\")"=w277) -> ("States Out"=w276:string)  [unwired: 14 in]
        }
        frame "UI: Cursor Set" {
          # "Argument"
          # "Set and Unset Cursor Busy.\n(Usage: \"UI: Cursor Set >> Busy|Idle\")"
          n132 = case shown="\"Busy\"" w280 {
            tunnel: w279 -> [w285 w287]
            tunnel: [w284 w286] -> w278
            frame "Idle", Default {
              n133 = call <vilib>:"Unset Busy.vi"("error in (no error)"=w285) -> ("error out"=w284:errorcluster)  [unwired: 10 in]
            }
            frame "Busy" {
              n134 = call <vilib>:"Set Busy.vi"("error in (no error)"=w287) -> ("error out"=w286:errorcluster)  [unwired: 9 in, 1 out]
            }
          }
          n135 = call <vilib>:"Add State(s) to Queue__JKI_lib_State_Machine.vi"("State(s) in (\"\")"=w283) -> ("States Out"=w282:string)  [unwired: 14 in]
        }
        frame "UI: Front Panel State" {
          # "Argument"
          # "Set Front Panel Open or Closed\n(Usage: \"UI: Front Panel State >> Open|Close\")"
          n136 = Unbundle By Name(w290) -> ("Core.Current VI Reference"=w289:refnum<vi>)
          n137 = case shown="\"Open\", Default" w288 {
            tunnel: w292 -> [w298 w311]
            tunnel: [w300 w312] -> w291
            tunnel: w289 -> [w299 w309]
            frame "Open", Default {
              n138 = property class="VI"(reference=w299, error in=w298) -> (reference out=w296:refnum<vi>, error out=w297:errorcluster, "Front Panel.Open"=w295:bool)
              n139 = case shown="True" w295 {
                tunnel: [w303 w306] -> w300
                tunnel: w297 -> [w302 w306]
                tunnel: w296 -> [w301 _]
                frame False {
                  n140 = invoke class="VI" method="FP.Open"(reference=w301, error in=w302, "Activate"=TRUE, "State"=T5."Standard") -> (error out=w303:errorcluster)  [unwired: 1 in, 4 out]
                }
                frame True {
                }
              }
            }
            frame "Close" {
              n141 = property class="VI"(reference=w309, error in=w311) -> (reference out=w308:refnum<vi>, error out=w310:errorcluster, "Front Panel.Open"=w307:bool)
              n142 = case shown="False" w307 {
                tunnel: [w313 w316] -> w312
                tunnel: w310 -> [w313 w315]
                tunnel: w308 -> [_ w314]
                frame False {
                }
                frame True {
                  n143 = invoke class="VI" method="FP.Close"(reference=w314, error in=w315) -> (error out=w316:errorcluster)  [unwired: 1 in, 2 out]
                }
              }
            }
          }
          n144 = call <vilib>:"Add State(s) to Queue__JKI_lib_State_Machine.vi"("State(s) in (\"\")"=w294) -> ("States Out"=w293:string)  [unwired: 14 in]
        }
        frame "---------- Macro ----------" {
          # "Do not put any code in this frame.\n(It is a separator no-op. You can make a copy of this frame to create a new Macro frame)"
          n145 = call <vilib>:"Add State(s) to Queue__JKI_lib_State_Machine.vi"("State(s) in (\"\")"=w320) -> ("States Out"=w319:string)  [unwired: 14 in]
        }
        frame "Macro: Initialize" {
          # "Initialization Macro\n(This is called once, when the VI starts)"
          n146 = call <vilib>:"Add State(s) to Queue__JKI_lib_State_Machine.vi"("State(s) in Front (\"\")"="Data: Initialize\nInitialize Core Data\n\nData: Run Edit VIs\nData: Create Data Queue\nData: 3D Initialize\n\nUI: Initialize\nUI: Front Panel State >> Open\nUI: Update Subpanel\nUI: Update AFM Subpanels\n\nLitho: Load SVG\nLitho: Load Background\nLitho: Update Information\nLitho: Order Data\nLitho: Refresh Render", "State(s) in (\"\")"=w325) -> ("States Out"=w324:string)  [unwired: 13 in]
        }
        frame "Macro: Exit" {
          # "Exit Macro\n(This is called once, when the VI exits)"
          n147 = Unbundle By Name(w326) -> ("Core.Close Panel on Exit?"=w332:bool)
          n148 = Select(t="UI: Front Panel State >> Close", s=w332, f="") -> (s? t:f=w329:string)
          n149 = call <vilib>:"Add State(s) to Queue__JKI_lib_State_Machine.vi"("State(s) in (\"\")"=w329, "State(s) at Back (\"\")"="Data: Cleanup\nExit") -> ("States Out"=w327:string)  [unwired: 13 in]
          n150 = call <vilib>:"Add State(s) to Queue__JKI_lib_State_Machine.vi"("State(s) in Front (\"\")"=w327, "State(s) in (\"\")"=w335) -> ("States Out"=w334:string)  [unwired: 13 in]
        }
        frame "---------- Litho ----------" {
          # "Template Separator\n(You can make a copy of, or modify, this frame)"
          n151 = call <vilib>:"Add State(s) to Queue__JKI_lib_State_Machine.vi"("State(s) in (\"\")"=w339) -> ("States Out"=w338:string)  [unwired: 14 in]
        }
        frame "Litho: Load SVG" {
          # "Check to see if specified file exists"
          # "Load SVG\nParses the SVG and stores the data obtained from it."
          n152 = local read "Inkscape File (.svg)"() -> (w346:path)
          n153 = call <vilib>:"Get File Extension.vi"("error in (no error)"=w344, "file"=w346) -> ("error out"=w343:errorcluster, "lowercase file extension"=w342:string, "dup file"=w345:path)  [unwired: 5 in, 2 out]
          n154 = case shown="Default" w342 {
            tunnel: w345 -> [_ w360]
            tunnel: w343 -> [w358 w359]
            tunnel: [w357 w360] -> w341
            tunnel: [w356 w359] -> w340
            frame Default {
              # "Change file to selected value"
              # "File doesnt exist: Have user select file."
              n155 = call "File Dialog"("prompt"="Choose an SVG file", "error in"=w358, "pattern (all files)"="*.svg") -> ("selected path"=w357:path, "error out"=w356:errorcluster)  [unwired: 9 in, 2 out]
            }
            frame "svg" {
              # "File exists: use it."
            }
          }
          n156 = call "SVG Parser.vi"("error in (no error)"=w340, "XML File Path"=w341) -> ("error out"=w351:errorcluster, "Parsing Data"=w350:T22, "Image Size"=w348:cluster{"Width":dbl, "Height":dbl})  [unwired: 1 in]
          n157 = local write "Inkscape File (.svg)"(w341) -> ()
          n158 = Bundle By Name(cluster=w349, "Parsing Data"=w350) -> (w347:T17)
          n159 = global write "Global Variables.vi" "Size"(w348) -> ()
          n160 = call <vilib>:"Add State(s) to Queue__JKI_lib_State_Machine.vi"("State(s) in (\"\")"=w353) -> ("States Out"=w352:string)  [unwired: 14 in]
        }
        frame "Litho: Load Background" {
          # "Check to see if specified file exists"
          # "Load Background\nLoads the background file into the images."
          n161 = local read "Background Image"() -> (w366:path)
          n162 = call <vilib>:"Get File Extension.vi"("error in (no error)"=w363, "file"=w366) -> ("error out"=w362:errorcluster, "lowercase file extension"=w364:string, "dup file"=w365:path)  [unwired: 5 in, 2 out]
          n163 = case shown="Default" w364 {
            tunnel: w362 -> [w382 w387]
            tunnel: [w384 w386] -> w361
            tunnel: [w385 w387] -> w368
            tunnel: w365 -> [_ w386]
            frame Default {
              # "Change file to selected value"
              # "File doesnt exist: Have user select file."
              n164 = call "File Dialog2"("prompt"="Choose an IBW file", "error in"=w382, "pattern (all files)"="*.ibw") -> ("selected path"=w384:path, "error out"=w385:errorcluster)  [unwired: 9 in, 2 out]
            }
            frame "ibw" {
              # "File exists: use it."
            }
          }
          n165 = local read "Page"() -> (w374:i32)
          n166 = call "Background.vi"("image data max"="image data max", "image data min"="image data min", "error in (no error)"=w368, "Page"=w374, "Image File Path"=w361) -> ("error out"=w377:errorcluster, "Background out"=w371:T2)  [unwired: 5 in]
          n167 = local write "Background Image"(w361) -> ()
          n168 = local write "Render"(w371) -> ()
          n169 = call "Imaq Create"("Image Name"="2D", "error in (no error)"=w377) -> ("New Image"=w378:T2, "error out"=w375:errorcluster)  [unwired: 3 in]
          n170 = call "IMAQ Copy"("error in (no error)"=w375, "Image Dst"=w378, "Image Src"=w371) -> ("error out"=w372:errorcluster, "Image Dst Out"=w373:T2)  [unwired: 3 in]
          n171 = call <vilib>:"Add State(s) to Queue__JKI_lib_State_Machine.vi"("State(s) in (\"\")"=w380) -> ("States Out"=w379:string)  [unwired: 14 in]
          n172 = local write "2D"(w373) -> ()
        }
        frame "Litho: Update Information" {
          # "Update the lithography data (toolpath)\nUses the parsing data and the properties of each pattern to generate the lithography data."
          n173 = Unbundle By Name(w388) -> ("Parsing Data"=w391:T18)
          n174 = local read "interpolation distance"() -> (w395:dbl)
          n175 = global read "Global Variables.vi" "Rectangle Properties"() -> (w390:T6[])
          n176 = global read "Global Variables.vi" "Path Properties"() -> (w389:T12[])
          n177 = global read "Global Variables.vi" "Funnel Properties"() -> (w397:T11[])
          n178 = call "Toolpath.vi"("interpolation distance"=w395, "Funnel Properties"=w397, "Parsing Data"=w391, "Path Properties"=w389, "Rectangle Properties"=w390) -> ("Estimated Time Required"=w396:timestamp, "Lithography Data"=w398:T19)  [unwired: 3 in]
          n179 = local write "Estimated Time\nfor Lithography"(w396) -> ()
          n180 = Bundle By Name(cluster=w388, "Lithography Data"=w398) -> (w394:T17)
          n181 = call <vilib>:"Add State(s) to Queue__JKI_lib_State_Machine.vi"("State(s) in Front (\"\")"="Driver: Update Controls" ("State(s) in Front (\"\")"), "State(s) in (\"\")"=w393) -> ("States Out"=w400:string)  [unwired: 13 in]
        }
        frame "Litho: Order Data" {
          # "Order the Patterns\nUses the ordering data to fix lithography data."
          n182 = Unbundle By Name(w402) -> ("Lithography Data"=w407:T19)
          n183 = control-ref of="Patterns (drag-and-drop reorder)"() -> (w406:refnum<vi>)
          n184 = call "Order Patterns.vi"("error in (no error)"=w401, "Lithography Data"=w407, "ListBox Reference in"=w406) -> ("error out"=w405:errorcluster, "Ordered Lithography Data"=w408:T19)  [unwired: 7 in]
          n185 = Bundle By Name(cluster=w402, "Lithography Data"=w408) -> (w403:T17)
          n186 = call <vilib>:"Add State(s) to Queue__JKI_lib_State_Machine.vi"("State(s) in Front (\"\")"="Driver: Update Controls" ("State(s) in Front (\"\")"), "State(s) in (\"\")"=w410) -> ("States Out"=w409:string)  [unwired: 13 in]
        }
        frame "Litho: Refresh Render" {
          # "Update the images\nUses the lithography data to update the images."
          n187 = Unbundle By Name(w413) -> ("Lithography Data"=w411:T19, "3D.Canvas"=w423:refnum<vi>)
          n188 = control-ref of="Voltage Mapping"() -> (w421:refnum<vi>)
          n189 = local read "Render"() -> (w420:T2)
          n190 = call "Image Generator.vi"("ColorRamp in"=w421, "Lithography Data"=w411, "error in (no error)"=w414, "Image Reference In"=w420) -> ("error out"=w419:errorcluster, "Image Reference Out"=w416:T2)  [unwired: 6 in]
          n191 = local write "Render"(w416) -> ()
          n192 = local read "2D"() -> (w415:T2)
          n193 = call "Convert IMAQ to LV Image.vi"("error in (no error)"=w419, "IMAQImage In (RGB 32)"=w415) -> ("error out"=w417:errorcluster, "Output Image"=w418:T15)  [unwired: 7 in, 1 out]
          n194 = call-poly <vilib>:"Apply Texture.vi"("error in (no error)"=w417, "Image Data"=w418, "Scene Object In"=w423) -> ("error out"=w422:errorcluster)  [unwired: 7 in, 1 out]
          n195 = invoke on="3D Picture" class="SceneGraphDisp (strict)" method="Redraw"(error in=w422) -> (error out=w412:errorcluster)  [unwired: 2 in, 2 out]
          n196 = call <vilib>:"Add State(s) to Queue__JKI_lib_State_Machine.vi"("State(s) in (\"\")"=w425) -> ("States Out"=w424:string)  [unwired: 14 in]
        }
        frame "---------- Driver ----------" {
          # "Template Separator\n(You can make a copy of, or modify, this frame)"
          n197 = call <vilib>:"Add State(s) to Queue__JKI_lib_State_Machine.vi"("State(s) in (\"\")"=w429) -> ("States Out"=w428:string)  [unwired: 14 in]
        }
        frame "Driver: Update Controls" {
          # "Driver is updated to reflect AFM type."
          n198 = Unbundle By Name(w437) -> ("Lithography Data"=w441:T19, "Data Queue"=w436:refnum<queue>)
          n199 = control-ref of="Abort"() -> (w434:refnum<vi>)
          n200 = control-ref of="Run 2"() -> (w432:refnum<vi>)
          n201 = control-ref of="Run"() -> (w433:refnum<vi>)
          n202 = property on="AFM Settings" class="SubPnl"() -> ("InsertedVI"=w442:refnum<vi>)  [unwired: 2 in, 2 out]
          n203 = control-ref of="Inkscape File (.svg)"() -> (w431:refnum<vi>)
          n204 = control-ref of="Background Image"() -> (w430:refnum<vi>)
          n205 = property on="Acquired Data" class="SubPnl"() -> ("InsertedVI"=w438:refnum<vi>)  [unwired: 2 in, 2 out]
          n206 = call "Set Driver Controls.vi"("Background Image"=w430, "Abort"=w434, "Inkscape File (.svg)"=w431, "Run"=w433, "error in (no error)"=w435, "Data Queue"=w436, "Lithography Data"=w441, "VI in"=w442) -> ()  [unwired: 2 in, 2 out]
          n207 = call "Set Driver Controls.vi"("Background Image"=w430, "Abort"=w434, "Inkscape File (.svg)"=w431, "Run"=w432, "Data Queue"=w436, "Lithography Data"=w441, "VI in"=w438) -> ("error out"=w440:errorcluster)  [unwired: 3 in, 1 out]
          n208 = Merge Errors(w440, w435) -> (w439:errorcluster)
          n209 = call <vilib>:"Add State(s) to Queue__JKI_lib_State_Machine.vi"("State(s) in (\"\")"=w444) -> ("States Out"=w443:string)  [unwired: 14 in]
        }
      }
      "Ready?" <- w5
    }
  }
